vi "_PC_Pub_ExpCondiValue_HV.vi"(2 "error in (no error)":errorcluster, 3 "expCondiVariant":variant) -> (0 "error out":errorcluster, 1 "d999Value":T1)   [LabVIEW 2018]
uses:
  RT/PublicSubVI/Ctl/_ctl_RT_D999_Format.ctl
  <vilib>/Utility/error.llb/Error Cluster From Error Code.vi
  <vilib>/ErrorRing/Error Ring.xnode
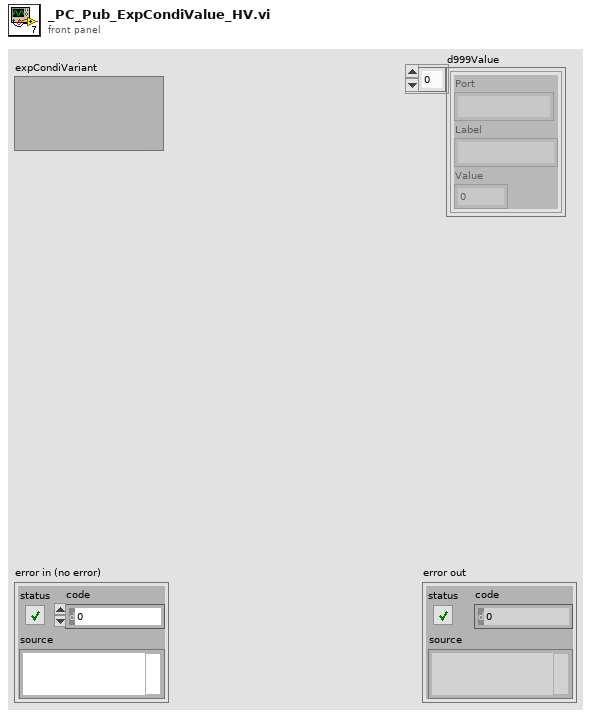
[diagram p1: front panel]
types:
  T1 = typedef "_ctl_RT_D999_Format.ctl" = cluster{"Port":string, "Label":string, "Value":dbl}[]
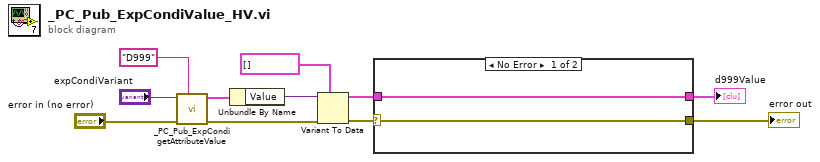
[diagram p0: block diagram]
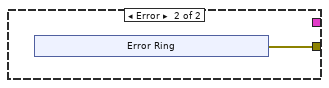
[diagram p2: hidden frame]
diagram:
  n1 = call "_PC_Pub_ExpCondi getAttributeValue.vi"("attrName"="D999", "error in (no error)"="error in (no error)", "expCondiVariant"="expCondiVariant") -> ("error out"=w8:errorcluster, "attrValue"=w11:cluster{"Label":string, "Value":variant})  [unwired: 7 in]
  n2 = Unbundle By Name(w11) -> ("Value"=w9:variant)
  n3 = Variant To Data(error in=w8, type=T1 [] ("Value"), Variant=w9) -> (data=w6:T1, error out=w7:errorcluster)
  n4 = case shown="No Error" w7 {
    selector: w7 -> [w12 _]
    tunnel: w6 -> [w13 _]
    tunnel: [w13 _] -> w1
    tunnel: [w12 w14] -> w4
    frame No Error {
    }
    frame Error {
      n5 = xnode "Error Ring"() -> ("error out"=w14:errorcluster)
    }
  }
  "d999Value" <- w1
  "error out" <- w4
